vi "Init Teller.vi"(6 "Teller Metadata":refnum<class "Teller Metadata.lvclass">, 9 "Relation":T1, 10 "Attributes":refnum<class "Attributes.lvclass">) -> (3 "Base Teller out":refnum<class "Base Teller.lvclass">)   [LabVIEW 2025, in "jettl.lvlib" / "Base Teller.lvlib" / "Base Teller.lvclass"]
uses:
  Base Teller.lvclass
  Relation.ctl
  Attributes/Attributes.lvclass
  Teller Metadata/Teller Metadata.lvclass
  Base Teller.lvclass/Base Teller.ctl
  jettl.lvlib
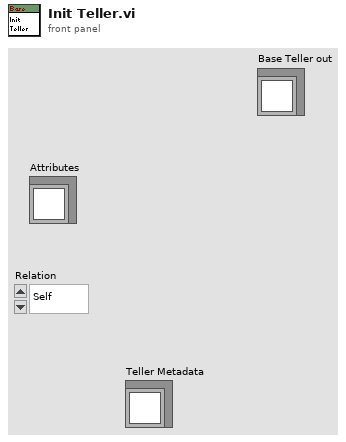
[diagram p1: front panel]
types:
  T1 = typedef "jettl.lvlib/Relation.ctl" = enum16{"Self", "Parent", "Child", "No Relation"}
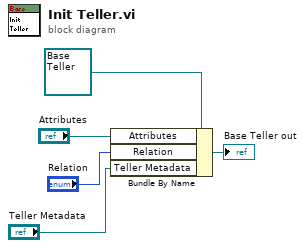
[diagram p0: block diagram]
diagram:
  n1 = Bundle By Name(cluster=refnum<class "Base Teller.lvclass"> refnum ("Base Sender out"), "Attributes"="Attributes", "Relation"="Relation", "Teller Metadata"="Teller Metadata") -> (→"Base Teller out":refnum<class "Base Teller.lvclass">)
